vi "FTW-CodeGen-Bounds.vi"(0 "State In":T1, 5 "XRef":refnum<vi>) -> (4 "Bounds":cluster{"Width":i32, "Height":i32})   [LabVIEW 2013, in "Featherweight.lvlib" / "FTW-SQLite-Fetch.xnode"]
uses:
  FTW-SQLite-Fetch.xnode
  FTW-CodeGen-State.ctl
panel:
  # "Inputs"
  # "Outputs"
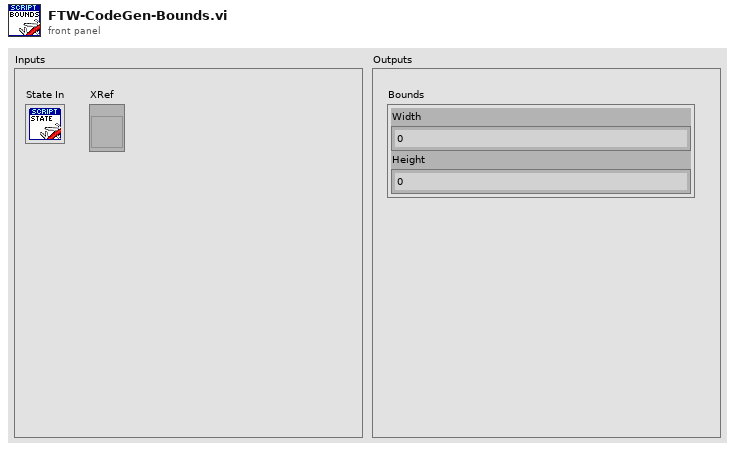
[diagram p1: front panel]
types:
  T1 = typedef "Featherweight.lvlib/FTW-SQLite-Fetch.xnode/FTW-CodeGen-State.ctl" = cluster{"Dummy":string}
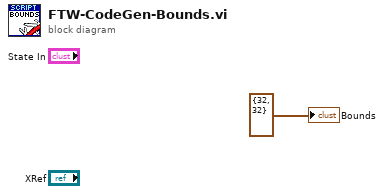
[diagram p0: block diagram]
diagram:
  "Bounds" <- cluster{"Width":i32, "Height":i32} {"Width"=32, "Height"=32} ("Bounds")
